vi "Autonomous.vi"   [LabVIEW 2025]
doc: "This VI starts when autonomous period begins, and will automatically be terminated when it ends. You can carry out timed or sensor driven operations directly to I/O or to subsystems without needing to return to the caller."
uses:
  <vilib>/Rock Robotics/WPI/ThirdParty/Phoenix-LabVIEW/Pigeon IMU/CTRE_PigeonIMU_TareType.ctl
  bb05fb8c-ae68-48c9-9160-d1d1c1cd9b74.vi
  <vilib>/Rock Robotics/WPI/Utilities/WPI_GetSetVariantRefNum.vi
  <vilib>/Rock Robotics/Network Tables/NT Read Number.vi
types:
  T1 = typedef "WPI_JoystickDevRef.ctl" = cluster{"Device":T2}
  T2 = typedef "WPI_JoystickDeviceEnum.ctl" = enum16{"USB 0", "USB 1", "USB 2", "USB 3", "USB 4", "USB 5"}
  T3 = typedef "CTRE_PigeonIMU_TareType.ctl" = u8
  T4 = typedef "Auto Data.ctl" = cluster{"Auto Data":cluster{"Velocities":T5[], "Positions":cluster{"x":dbl, "y":dbl, "th":dbl}[], "Command Info":cluster{dbl, "Command out":cluster{"Name":string, "vi reference":refnum<vi>, i32[], variant[]}}[], "Zero Velocity?":bool[], "Zero Translational Velocity?":bool[], "Current Limit":dbl, "Correct at Beginning of Path":bool}[], "Number of Remaining Auto Paths":dbl}
  T5 = typedef "Robot Velocities.ctl" = cluster{"X Velocity":dbl, "Y Velocity":dbl, "Rotational \nVelocity":dbl}
  T6 = cluster{"Velocities":T5[], "Positions":cluster{"x":dbl, "y":dbl, "th":dbl}[], "Command Info":cluster{dbl, "Command out":cluster{"Name":string, "vi reference":refnum<vi>, i32[], variant[]}}[], "Zero Velocity?":bool[], "Zero Translational Velocity?":bool[], "Current Limit":dbl, "Correct at Beginning of Path":bool}[]
  T7 = cluster{"Velocities":T5[], "Positions":cluster{"x":dbl, "y":dbl, "th":dbl}[], "Command Info":cluster{dbl, "Command out":cluster{"Name":string, "vi reference":refnum<vi>, i32[], variant[]}}[], "Zero Velocity?":bool[], "Zero Translational Velocity?":bool[], "Current Limit":dbl, "Correct at Beginning of Path":bool}
  T8 = typedef "CTRE_PigeonIMU_DeviceRef.ctl" = cluster{"DeviceStatus":errorcluster, "Device Number":u8, "Type":T9, "Device ID":u32, "Handle":u64, "UsageFrame":u32, "Library Path":path}
  T9 = typedef "CTRE_PigeonIMU_ConnectionType.ctl" = u32
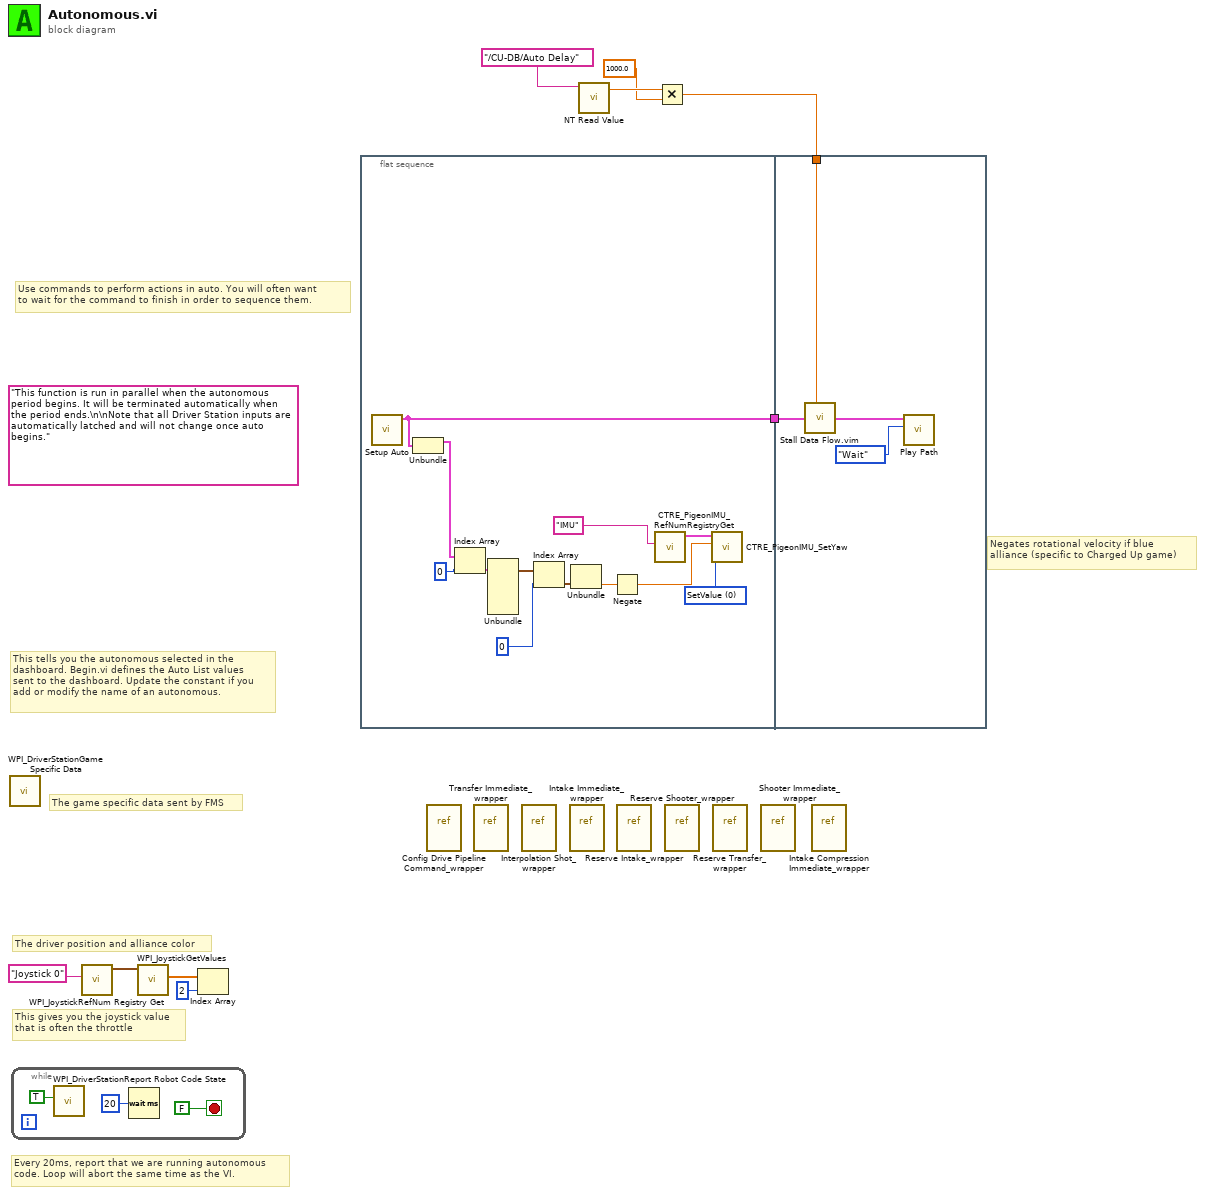
[diagram p0: block diagram]
diagram:
  (unwired) "This function is run in parallel when the autonomous period begins. It will be terminated automatically when the period ends.\n\nNote that all Driver Station inputs are automatically latched and will not change once auto begins."
  # "Negates rotational velocity if blue alliance (specific to Charged Up game)"
  # "The game specific data sent by FMS"
  # "This tells you the autonomous selected in the \ndashboard. Begin.vi defines the Auto List values\nsent to the dashboard. Update the constant if you\nadd or modify the name of an autonomous."
  # "Every 20ms, report that we are running autonomous\ncode. Loop will abort the same time as the VI."
  # "This gives you the joystick value\nthat is often the throttle"
  # "Use commands to perform actions in auto. You will often want\nto wait for the command to finish in order to sequence them."
  # "The driver position and alliance color"
  n1 = call <vilib>:"WPI_DriverStationGame Specific Data.vi"() -> ()  [unwired: 11 in, 1 out]
  n2 = while {
    stop <- FALSE stop-if-true
    n3 = call <vilib>:"WPI_DriverStationReport Robot Code State.vi"("Autonomous"=TRUE) -> ()  [unwired: 10 in, 1 out]
    n4 = Wait (ms)(milliseconds to wait=u32 20) -> ()  [unwired: 1 out]
  }
  n5 = call <vilib>:"WPI_JoystickRefNum Registry Get.vi"("refnum name"="Joystick 0") -> ("JoystickDevRef"=w8:T1)  [unwired: 1 in, 9 out]
  n6 = call <vilib>:"WPI_JoystickGetValues.vi"("JoystickDevRef"=w8) -> ("Axes"=w7:dbl[])  [unwired: 6 in, 4 out]
  n7 = Index Array(array=w7, index=2) -> ()  [unwired: 1 out]
  n8 = flat-sequence {
    tunnel: [w19] -> w5
    tunnel: w5 -> [w26]
    tunnel: w1 -> [w27]
    frame #0 {
      w15 = T3 0 items=["SetValue"=0, "AddOffset"=1, "MatchCompass"=2, "SetOffset"=255] ("TareType (SetValue)")
      n9 = call "Setup Auto.vi"() -> ("Auto Data"=w19:T4)  [unwired: 11 in]
      n10 = Unbundle(w19) -> ("Auto Data"=w17:T6)  [unwired: 1 out]
      n11 = Index Array(array=w17, index=0 ("index (row)")) -> (element=w22:T7)
      n12 = Unbundle(w22) -> ("Positions"=w16:cluster{"x":dbl, "y":dbl, "th":dbl}[])  [unwired: 6 out]
      n13 = Index Array(array=w16, index=0 ("index (row)")) -> (element=w24:cluster{"x":dbl, "y":dbl, "th":dbl})
      n14 = Unbundle(w24) -> ("th"=w18:dbl)  [unwired: 2 out]
      n15 = Negate(x=w18) -> (-x=w13:dbl)
      n16 = call <vilib>:"CTRE_PigeonIMU_RefNumRegistryGet.vi"("refnum name"="IMU") -> ("PigeonIMUDevRef"=w14:T8)  [unwired: 9 in, 1 out]
      n17 = call <vilib>:"CTRE_PigeonIMU_SetYaw.vi"("TareType (SetValue)"=w15, "Value"=w13, "PigeonIMUDevRef"=w14) -> ()  [unwired: 7 in, 2 out]
    }
    frame #1 {
      n18 = call "Stall Data Flow.vim"("value in"=w26, "milliseconds to wait"=w27) -> ("value out"=w25:T4)  [unwired: 1 out]
      n19 = call "Play Path.vi"("Synchronization"=enum16{"Start", "Wait"}."Wait", "Auto Data"=w25) -> ()  [unwired: 9 in, 1 out]
    }
  }
  n20 = vi-ref "Config Drive Pipeline Command_wrapper.vi"() -> ()  [unwired: 1 out]
  n21 = vi-ref "Transfer Immediate_wrapper.vi"() -> ()  [unwired: 1 out]
  n22 = vi-ref "Interpolation Shot_wrapper.vi"() -> ()  [unwired: 1 out]
  n23 = vi-ref "Intake Immediate_wrapper.vi"() -> ()  [unwired: 1 out]
  n24 = call-poly <vilib>:"NT Read Value.vi"("name"="/CU-DB/Auto Delay") -> ("value"=w3:dbl)  [unwired: 8 in, 2 out]
  n25 = vi-ref "Reserve Intake_wrapper.vi"() -> ()  [unwired: 1 out]
  n26 = Multiply(x=w3, y=1000.0) -> (x*y=w1:dbl)
  n27 = vi-ref "Reserve Shooter_wrapper.vi"() -> ()  [unwired: 1 out]
  n28 = vi-ref "Reserve Transfer_wrapper.vi"() -> ()  [unwired: 1 out]
  n29 = vi-ref "Shooter Immediate_wrapper.vi"() -> ()  [unwired: 1 out]
  n30 = vi-ref "Intake Compression Immediate_wrapper.vi"() -> ()  [unwired: 1 out]
